vi "read_params.vi"(8 "error in (no error)":errorcluster, 11 "CategoricalNB in":refnum<class "CategoricalNB.lvclass">) -> (0 "error out":errorcluster, 2 "params":T1={"alpha"=1.0, "fit_prior"=TRUE, "class_prior"={"class_prior_type"="None", "class_prior_list"=[]}, "min_categories"={"min_categories_type"="None", "min_categories_list"=[]}}, 3 "CategoricalNB out":refnum<class "CategoricalNB.lvclass">)   [LabVIEW 2020, in "CategoricalNB.lvclass"]
uses:
  CategoricalNB.lvclass
  Controls/categorical_nb_params.ctl
  CategoricalNB.lvclass/CategoricalNB.ctl
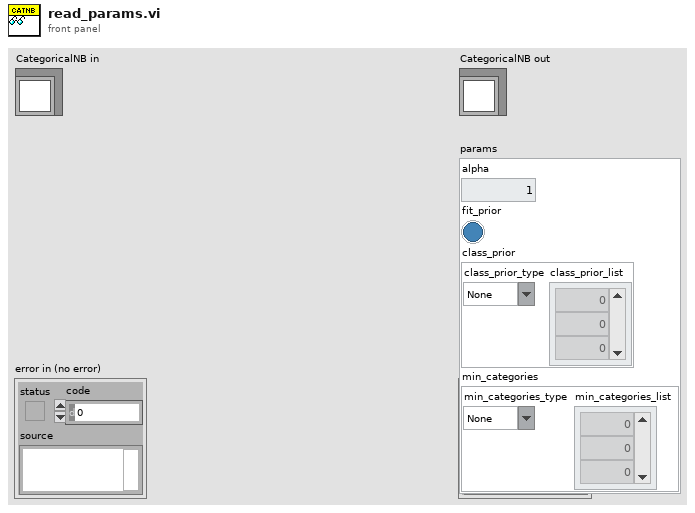
[diagram p1: front panel]
types:
  T1 = typedef "categorical_nb_params.ctl" = cluster{"alpha":dbl, "fit_prior":bool, "class_prior":cluster{"class_prior_type":string, "class_prior_list":dbl[]}, "min_categories":cluster{"min_categories_type":string, "min_categories_list":dbl[]}}
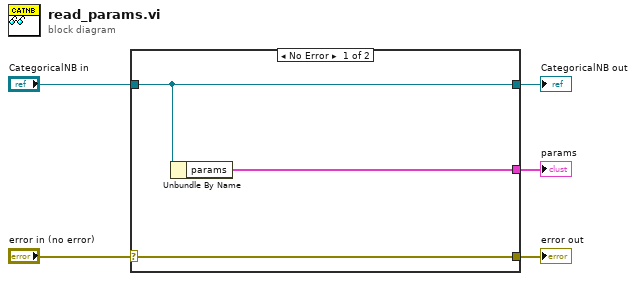
[diagram p0: block diagram]
diagram:
  n1 = case shown="No Error" "error in (no error)" {
    selector: "error in (no error)" -> [w8 w9]
    tunnel: [w8 w9] -> w4
    tunnel: [w7 w10] -> w2
    tunnel: "CategoricalNB in" -> [w7 w10]
    tunnel: [w6 _] -> w1
    frame No Error {
      n2 = Unbundle By Name(w7) -> ("params"=w6:T1)
    }
    frame Error {
    }
  }
  "error out" <- w4
  "CategoricalNB out" <- w2
  "params" <- w1
